vi "NIDCPower_channel_ganging - configure current limit.vi"(7 "Limit Symmetry":i32(ring)=1 items=["Symmetric", "Asymmetric"], 8 "error in (no error)":errorcluster, 9 "Current limit/hi":dbl format="%#.6p", 10 "Current limit lo":dbl format="%#.6p", 11 "Ganged Session In":T1={"Ganged Config"=enum."Parallel", "Session List"=[], "Session Mode"=[], "Channel"=[]}) -> (0 "error out":errorcluster, 3 "Ganged Session Out":T1)   [LabVIEW 2021]
uses:
  ctl/NIDCPower_channel_ganging - ctl - ganged session.ctl
  ctl/NIDCPower_channel_ganging - ctl - ganged config.ctl
  ctl/NIDCPower_channel_ganging - ctl - channel mode.ctl
panel:
  in  "Channel":string="0"
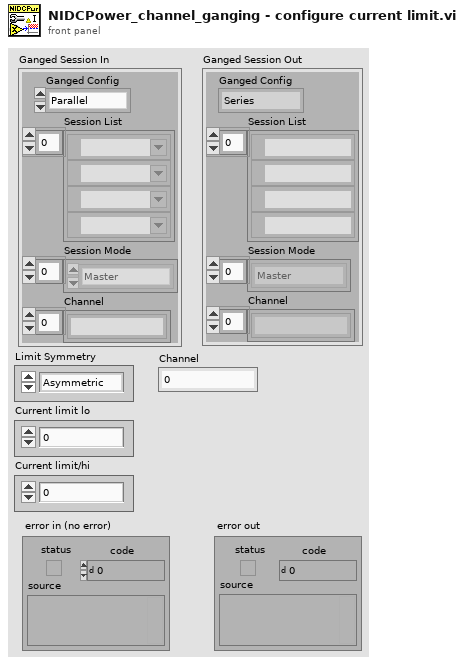
[diagram p1: front panel]
types:
  T1 = typedef "NIDCPower_channel_ganging - ctl - ganged session.ctl" = cluster{"Ganged Config":T2, "Session List":refnum<k15>[], "Session Mode":T3[], "Channel":string[]}
  T2 = typedef "NIDCPower_channel_ganging - ctl - ganged config.ctl" = enum32{"Series", "Parallel", "Manual"}
  T3 = typedef "NIDCPower_channel_ganging - ctl - channel mode.ctl" = enum32{"Master", "Slave", "Slave - Inverted"}
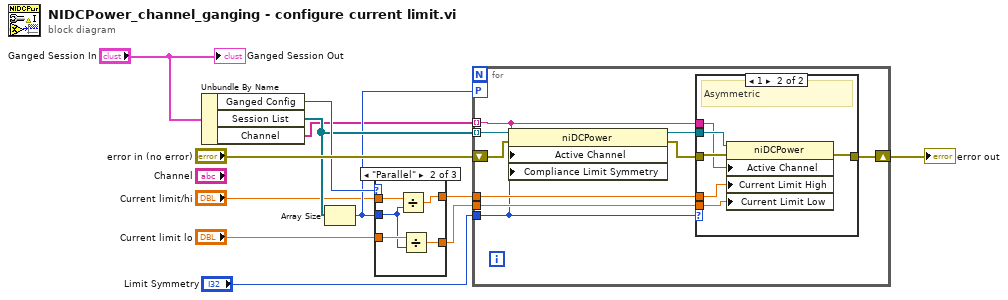
[diagram p0: block diagram]
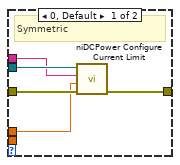
[diagram p4: hidden frame]
diagram:
  n1 = Unbundle By Name("Ganged Session In") -> ("Ganged Config"=w10:T2, "Session List"=w8:refnum<k15>[], "Channel"=w1:string[])
  n2 = Array Size(array=w8) -> (size(s)=w6:i32)
  n3 = case shown="\"Parallel\"" w10 {
    tunnel: w6 -> [_ w15 _]
    tunnel: "Current limit/hi" -> [w14 w19 w21]
    tunnel: [w14 w18 w21] -> w7
    tunnel: "Current limit lo" -> [w13 w17 w20]
    tunnel: [w13 w16 w20] -> w2
    frame "Series" {
    }
    frame "Parallel" {
      n4 = Divide(x=w19, y=w15) -> (x/y=w18:dbl)
      n5 = Divide(x=w17, y=w15) -> (x/y=w16:dbl)
    }
    frame "Manual" {
    }
  }
  n6 = for {
    shift-right: [w29] -> w11
    shift-left: "error in (no error)" -> [w24]
    tunnel: w8 -> [w27] mode=indexing
    tunnel: w7 -> [w30]
    workers-P: w6 -> [_]
    tunnel: "Limit Symmetry" -> [w23]
    tunnel: w2 -> [w28]
    tunnel: w1 -> [w22] mode=indexing
    n7 = property class="niDCPower"(reference=w27, error in=w24, "Active Channel"=w22, "Compliance Limit Symmetry"=w23) -> (reference out=w26:refnum<k15>, error out=w25:errorcluster)
    n8 = case shown="1" w23 {
      tunnel: w25 -> [w35 w39]
      tunnel: w26 -> [w34 w40]
      tunnel: w30 -> [w33 w37]
      tunnel: [w32 w41] -> w29
      tunnel: w28 -> [_ w38]
      tunnel: w22 -> [w31 w36]
      frame 0, Default {
        # "Symmetric"
        n9 = call <instrlib>:"niDCPower Configure Current Limit.vi"("error in (no error)"=w35, "current limit"=w33, "channel name"=w31, "instrument handle"=w34) -> ("error out"=w32:errorcluster)  [unwired: 6 in, 1 out]
      }
      frame 1 {
        # "Asymmetric"
        n10 = property class="niDCPower"(reference=w40, error in=w39, "Active Channel"=w36, "Current Limit High"=w37, "Current Limit Low"=w38) -> (error out=w41:errorcluster)  [unwired: 1 out]
      }
    }
  }
  "error out" <- w11
  "Ganged Session Out" <- "Ganged Session In"
